vi "fgv_vlp16_inrange.vi"(8 "error in":errorcluster) -> (0 "error out":errorcluster, 3 "data":T1(array[cluster]))   [LabVIEW 2019]
uses:
  Ctrl/vlp-16 cmd.ctl
  Ctrl/obstacle_info.ctl
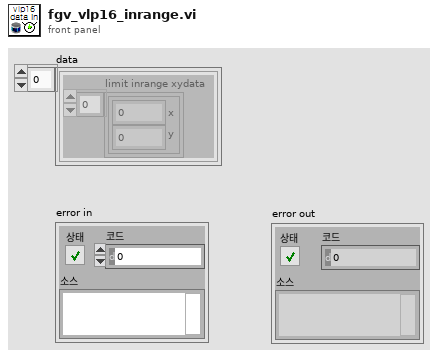
[diagram p1: front panel]
types:
  T1 = cluster{"limit inrange xydata":cluster{"x":dbl, "y":dbl}[]}[]
  T2 = typedef "obstacle_info.ctl" = enum16{"init", "read", "obstacle status in", "write limit", "inrange pt-n"}
  T3 = typedef "vlp-16 cmd.ctl" = enum16{"write all data", "write xyz data", "read"}
  T4 = cluster{"h range":cluster{i16, i16}, "v range":cluster{i8, i8}}
  T5 = cluster{"limit inrange xydata":cluster{"x":dbl, "y":dbl}[]}
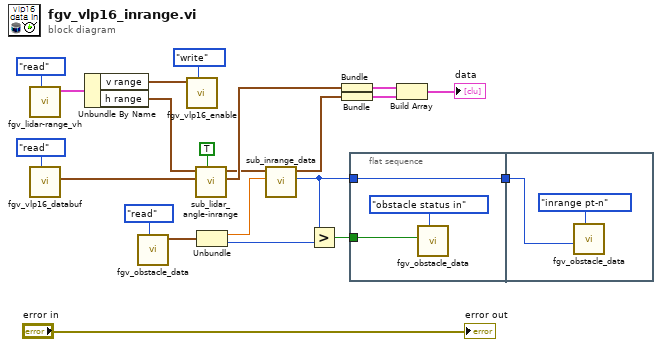
[diagram p0: block diagram]
diagram:
  n1 = call "fgv_lidar-range_vh.vi"("cmd"=enum16{"read", "write"}."read") -> ("VLP16 cfg out"=w10:T4)  [unwired: 10 in]
  n2 = call "fgv_vlp16_databuf.vi"("cmd"=vlp-16_cmd."read") -> ("xyz_data_out"=w20:cluster{"x":dbl, "y":dbl, "z":dbl}[])  [unwired: 8 in, 2 out]
  n3 = Unbundle By Name(w10) -> ("v range"=w13:cluster{i8, i8}, "h range"=w12:cluster{i16, i16})
  n4 = call "fgv_obstacle_data.vi"("cmd"=obstacle_info."read") -> ("limit out"=w16:cluster{"RL range":dbl, "Point limit":u16})  [unwired: 7 in, 3 out]
  n5 = call "fgv_vlp16_enable.vi"("cmd"=enum16{"init", "read", "write"}."write", "v range"=w13) -> ()  [unwired: 9 in, 1 out]
  n6 = call "sub_lidar_angle-inrange.vi"("3d"=TRUE, "3D data"=w20, "h range"=w12) -> ("xydata"=w22:cluster{"x":dbl, "y":dbl}[], "Array out"=w21:cluster{"x":dbl, "y":dbl}[])  [unwired: 6 in, 1 out]
  n7 = Unbundle(w16) -> ("RL range"=w19:dbl, "Point limit"=w1:u16)
  n8 = call "sub_inrange_data.vi"("limit"=w19, "xy_lidar data"=w21) -> ("limit point out"=w2:u16, "limit inrange xydata"=w17:cluster{"x":dbl, "y":dbl}[])  [unwired: 7 in, 1 out]
  n9 = Greater?(x=w2, y=w1) -> (0:w3:bool)
  n10 = Bundle("xydata"=w22) -> (w14:cluster{"xydata":cluster{"x":dbl, "y":dbl}[]})  [unwired: 1 in]
  n11 = Bundle("limit inrange xydata"=w17) -> (w18:T5)  [unwired: 1 in]
  n12 = flat-sequence {
    tunnel: w3 -> [w24]
    tunnel: [w23] -> w4
    tunnel: w2 -> [w23]
    tunnel: w4 -> [w26]
    frame #0 {
      n13 = call "fgv_obstacle_data.vi"("cmd"=obstacle_info."obstacle status in", "obstacle in"=w24) -> ()  [unwired: 6 in, 4 out]
    }
    frame #1 {
      n14 = call "fgv_obstacle_data.vi"("cmd"=obstacle_info."inrange pt-n", "inrange pt-n"=w26) -> ()  [unwired: 6 in, 4 out]
    }
  }
  n15 = Build Array(w14, w18) -> (→"data":T1)
  "error out" <- "error in"
